vi "ConfigAndGrab.vi"() -> ()   [LabVIEW 2012]
uses:
  <vilib>/userDefined/High Color/IMAQdx.ctl
  <vilib>/vision/driver/IMAQdx.llb/IMAQdx Buffer Number Mode.ctl
  <vilib>/vision/driver/NI_Vision_Acquisition_Software.lvlib
  <resource>/objmgr/imaqdx.rc
panel:
  out "DeviceModelName":string
  in  "OffsetY":i64=100
  in  "Height":i64=600
  in  "OffsetX":i64=200
  in  "Width":i64=800
  in  "ExposureTime":dbl=850.5
  in  "Camera Name":T1
  out "Frame Rate":dbl(knob) scale=0.0..100.0 scale format="%.1f"
  out "Buffer Number":u32
  out "Image":T2(plugin-control)
  in  "stop":bool
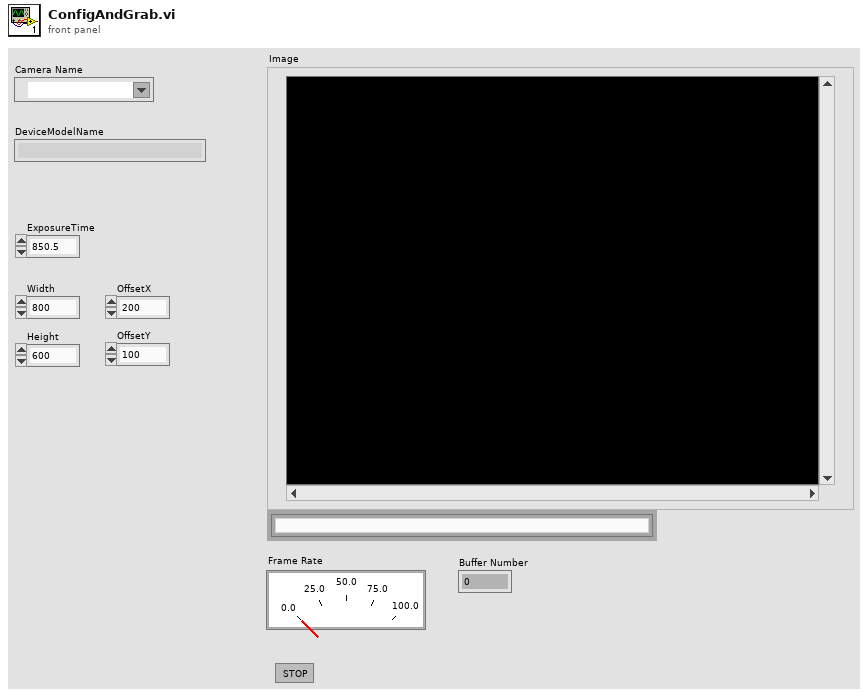
[diagram p1: front panel]
types:
  T1 = typedef "IMAQdx.ctl" = refnum<k21>
  T2 = typedef "IMAQ Image.ctl" = refnum<image>
  T3 = typedef "NI_Vision_Acquisition_Software.lvlib/IMAQdx Buffer Number Mode.ctl" = enum32{"Next", "Last", "Buffer Number"}
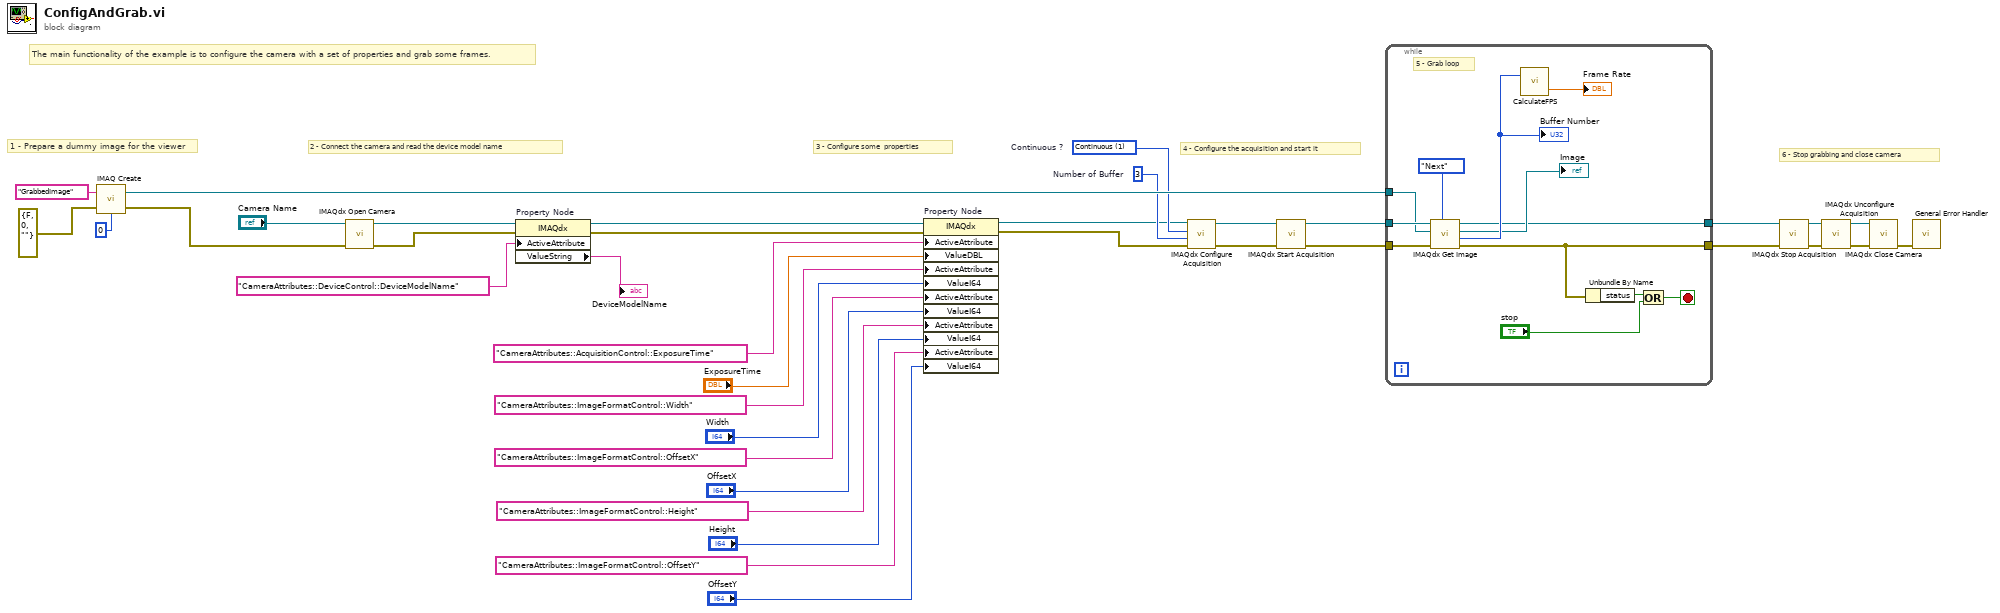
[diagram p0: block diagram]
diagram:
  w19 = u32 3  # Number of Buffer
  w18 = u32 1 items=["One Shot", "Continuous"]  # Continuous ?
  # "The main functionality of the example is to configure the camera with a set of properties and grab some frames."
  # "6 - Stop grabbing and close camera"
  # "4 - Configure the acquisition and start it"
  # "3 - Configure some  properties"
  # "2 - Connect the camera and read the device model name"
  # "1 - Prepare a dummy image for the viewer"
  n1 = call "IMAQ Create"("Image Name"="GrabbedImage", "Image Type"=0, "error in (no error)"=errorcluster {"status"=FALSE, "code"=0, "source"=""}) -> ("New Image"=w22:T2, "error out"=w23:errorcluster)  [unwired: 1 in, 1 out]
  n2 = call <vilib>:"IMAQdx Open Camera.vi"("error in"=w23, "Session In"="Camera Name") -> ("error out"=w4:errorcluster, "Session Out"=w20:T1)  [unwired: 8 in]
  n3 = property on="Property Node" class="IMAQdx"(reference=w20, error in=w4, "ActiveAttribute"="CameraAttributes::DeviceControl::DeviceModelName") -> (reference out=w5:T1, error out=w3:errorcluster, "ValueString"=→"DeviceModelName":string)
  n4 = property on="Property Node" class="IMAQdx"(reference=w5, error in=w3, "ActiveAttribute"="CameraAttributes::AcquisitionControl::ExposureTime", "ValueDBL"="ExposureTime", "ActiveAttribute"="CameraAttributes::ImageFormatControl::Width", "ValueI64"="Width", "ActiveAttribute"="CameraAttributes::ImageFormatControl::OffsetX", "ValueI64"="OffsetX", "ActiveAttribute"="CameraAttributes::ImageFormatControl::Height", "ValueI64"="Height", "ActiveAttribute"="CameraAttributes::ImageFormatControl::OffsetY", "ValueI64"="OffsetY") -> (reference out=w17:T1, error out=w16:errorcluster)
  n5 = call <vilib>:"IMAQdx Configure Acquisition.vi"("error in"=w16, "Number of Buffers"=w19, "Continuous?"=w18, "Session In"=w17) -> ("error out"=w37:errorcluster, "Session Out"=w36:T1)  [unwired: 6 out]
  n6 = call <vilib>:"IMAQdx Start Acquisition.vi"("error in"=w37, "Session In"=w36) -> ("error out"=w35:errorcluster, "Session Out"=w34:T1)  [unwired: 8 out]
  n7 = while {
    tunnel: w35 -> [w48]
    tunnel: w34 -> [w49]
    tunnel: w22 -> [w44]
    tunnel: [w40] -> w28
    tunnel: [w39] -> w27
    stop <- w41 stop-if-true
    # "5 - Grab loop"
    n8 = call <vilib>:"IMAQdx Get Image.vi"("Buffer Number Mode (Next)"=IMAQdx_Buffer_Number_Mode."Next", "error in"=w48, "Image In"=w44, "Session In"=w49) -> ("error out"=w40:errorcluster, "Buffer Number Out"=w45:u32, "Image Out"=→"Image":T2, "Session Out"=w39:T1)  [unwired: 4 in]
    "Buffer Number" <- w45
    n9 = call <userlib>:"CalculateFPS.vi"("buffer number"=w45) -> ("processed FPS"=→"Frame Rate":dbl)  [unwired: 2 out]
    n10 = Unbundle By Name(w40) -> ("status"=w42:bool)
    n11 = Or(x=w42, y="stop") -> (x .or. y?=w41:bool)
  }
  n12 = call <vilib>:"IMAQdx Stop Acquisition.vi"("error in"=w28, "Session In"=w27) -> ("error out"=w32:errorcluster, "Session Out"=w31:T1)  [unwired: 8 out]
  n13 = call <vilib>:"IMAQdx Unconfigure Acquisition.vi"("error in"=w32, "Session In"=w31) -> ("error out"=w29:errorcluster, "Session Out"=w30:T1)  [unwired: 8 out]
  n14 = call <vilib>:"IMAQdx Close Camera.vi"("error in"=w29, "Session In"=w30) -> ("error out"=w33:errorcluster)  [unwired: 9 out]
  n15 = call <vilib>:"General Error Handler.vi"("error in (no error)"=w33) -> ()  [unwired: 1 in, 14 out]
